vi "HPRF Signal Conditioner.vi"(7 "Signals":waveform(dbl)[](array[waveform]), 11 "error in (no error)":errorcluster) -> (8 "Condintioned Signals":waveform(dbl)[](array[waveform]), 15 "error out":errorcluster)   [LabVIEW 2013]
uses:
  <vilib>/Analysis/2dsp.llb/Real FFT.vi
  <vilib>/Waveform/WDTOps.llb/WDT Waveform Duration DBL.vi
  <vilib>/measure/maresamp.llb/Resample N Waveforms (single shot).vi
  <vilib>/measure/maresamp.llb/Resample Waveform (single shot).vi
  <vilib>/Waveform/WDTOps.llb/WDT Get Waveform Subset DBL.vi
  <vilib>/measure/NI_MAPro.lvlib
  <vilib>/Analysis/NI_AALPro.lvlib
panel:
  out "Input Signals":waveform(dbl)[](graph)
  out "Conditioned Signal":waveform(dbl)[](graph)
  out "FFT Imag":dbl[][](graph)
  out "FFT Real":dbl[][](graph)
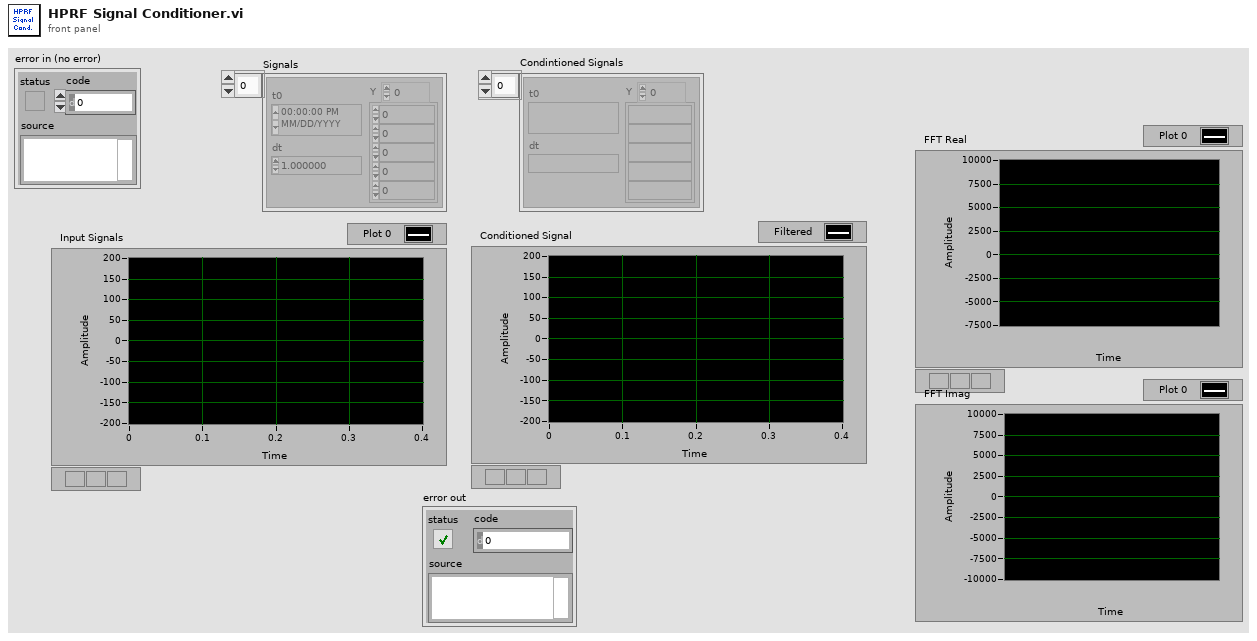
[diagram p1: front panel]
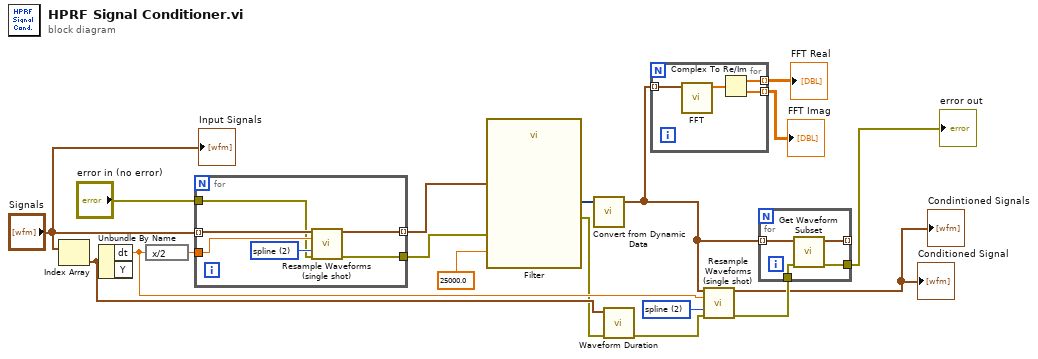
[diagram p0: block diagram]
diagram:
  w11 = u16 2 items=["coerce", "linear", "spline", "FIR filter"] ("interpolation mode")
  n1 = Index Array(array="Signals") -> (element=w6:waveform(dbl))  [unwired: 1 in]
  n2 = Unbundle By Name(w6) -> ("dt"=w10:dbl)  [unwired: 1 out]
  n3 = expression code="x/2"(w10) -> (w13:dbl)
  n4 = for {
    tunnel: [w24] -> w18 mode=indexing
    tunnel: "Signals" -> [w22] mode=indexing
    tunnel: w13 -> [w21]
    tunnel: [w20] -> w9
    tunnel: "error in (no error)" -> [w19]
    w23 = u16 2 items=["coerce", "linear", "spline", "FIR filter"] ("interpolation mode")
    n5 = call-poly <vilib>:"Resample Waveforms (single shot).vi"("waveform in"=w22, "dt"=w21, "interpolation mode"=w23, "error in (no error)"=w19) -> ("resampled waveform out"=w24:waveform(dbl), "error out"=w20:errorcluster)  [unwired: 8 in, 2 out]
  }
  n6 = call "Filter"("error in (no error)"=w9, "Lower Cut-Off"=25000.0, "Signal"=w18) -> ("error out"=w5:errorcluster, "Filtered Signal"=w16:dynamicdata)  [unwired: 7 in]
  n7 = call "Convert from Dynamic Data"("Dynamic Data Type"=w16) -> ("Array of Waveform"=w2:waveform(dbl)[])  [unwired: 3 in]
  n8 = call-poly <vilib>:"Waveform Duration.vi"("error in (no error)"=w5, "waveform in"=w6) -> ("error out"=w4:errorcluster)  [unwired: 7 in, 2 out]
  n9 = for {
    tunnel: w2 -> [w27] mode=indexing
    tunnel: [w26] -> w15 mode=indexing
    tunnel: [w25] -> w14 mode=indexing
    n10 = call-poly <vilib>:"FFT.vi"("X"=w27) -> ("FFT {X}"=w28:cdb[])  [unwired: 9 in, 1 out]
    n11 = Complex To Re/Im(x + iy=w28) -> (x=w26:dbl[], y=w25:dbl[])
  }
  "FFT Real" <- w15
  "FFT Imag" <- w14
  n12 = call-poly <vilib>:"Resample Waveforms (single shot).vi"("waveforms in"=w2, "dt"=w10, "interpolation mode"=w11, "error in (no error)"=w4) -> ("resampled waveforms out"=→"Conditioned Signal" →"Condintioned Signals":waveform(dbl)[], "error out"=w8:errorcluster)  [unwired: 8 in, 2 out]
  n13 = for {
    tunnel: w2 -> [w32] mode=indexing
    tunnel: [w31] -> _ mode=indexing
    tunnel: w8 -> [w30]
    tunnel: [w29] -> w7
    n14 = call-poly <vilib>:"Get Waveform Subset.vi"("error in (no error)"=w30, "waveform in"=w32) -> ("error out"=w29:errorcluster, "waveform out"=w31:waveform(dbl))  [unwired: 4 in, 2 out]
  }
  "error out" <- w7
  "Input Signals" <- "Signals"
